vi "AHRead2.vi"(8 "error in (no error)":errorcluster) -> (0 "error out":errorcluster, 1 "frequency":dbl, 2 "loss":dbl=nan format="%.7f", 3 "capacitance":dbl=nan format="%.7f")   [LabVIEW 2009]
uses:
  <instrlib>/Andeen-Hagerling 2550/Andeen-Hagerling 2550.lvlib
panel:
  out "Loss Chart":dbl(graph)
  out "Cap Chart":dbl(graph)
  out "Vexc":dbl=nan format="%.7f"
  out "out string":string
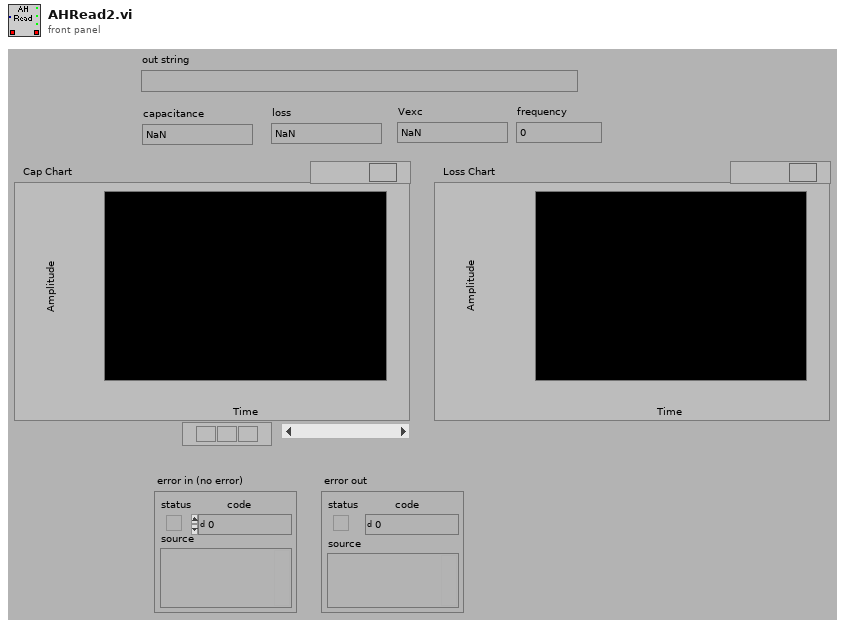
[diagram p1: front panel]
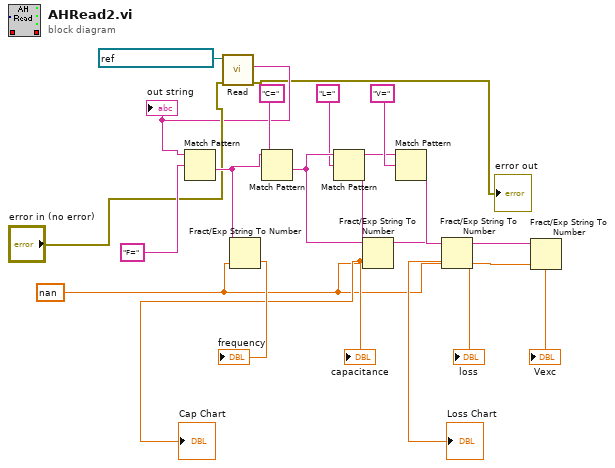
[diagram p0: block diagram]
diagram:
  w5 = nan ("default (0 dbl)")
  n1 = call <instrlib>:"Read.vi"("error in"="error in (no error)", "VISA resource name"=refnum<visa-resource-name> "GPIB0::28::INSTR") -> ("error out"=→"error out":errorcluster, "Message"=w2:string)  [unwired: 6 in, 2 out]
  "out string" <- w2
  n2 = Match Pattern(string=w2, regular expression="F=") -> (after substring=w9:string)  [unwired: 1 in, 3 out]
  n3 = Fract/Exp String To Number(string=w9, default (0 dbl)=w5) -> (number=→"frequency":dbl)  [unwired: 2 in, 1 out]
  n4 = Match Pattern(string=w9, regular expression="C=") -> (after substring=w16:string)  [unwired: 1 in, 3 out]
  n5 = Match Pattern(string=w16, regular expression="L=") -> (after substring=w12:string)  [unwired: 1 in, 3 out]
  n6 = Fract/Exp String To Number(string=w16, default (0 dbl)=w5) -> (number=→"capacitance" →"Cap Chart":dbl)  [unwired: 2 in, 1 out]
  n7 = Match Pattern(string=w12, regular expression="V=") -> (after substring=w14:string)  [unwired: 1 in, 3 out]
  n8 = Fract/Exp String To Number(string=w12, default (0 dbl)=w5) -> (number=→"loss" →"Loss Chart":dbl)  [unwired: 2 in, 1 out]
  n9 = Fract/Exp String To Number(string=w14, default (0 dbl)=w5) -> (number=→"Vexc":dbl)  [unwired: 2 in, 1 out]
